vi "core_h5_write_array_3d.vi"(4 "dim3 (index)":string="index", 6 "dim2 (index)":string="index", 7 "dataset name":string, 8 "error in (no error)":errorcluster, 9 "dim1 (index)":string="index", 10 "units (au)":string="au", 11 "h5 obj ref":i32) -> (0 "error out":errorcluster, 3 "h5 obj ref":i32)   [LabVIEW 2015]
uses:
  <vilib>/addons/h5labview2/base/lib_path.vi
  <vilib>/addons/h5labview2/base/H5Equery.vi
  <vilib>/addons/h5labview2/attrib/H5Awrite.llb/H5Awrite.xnode
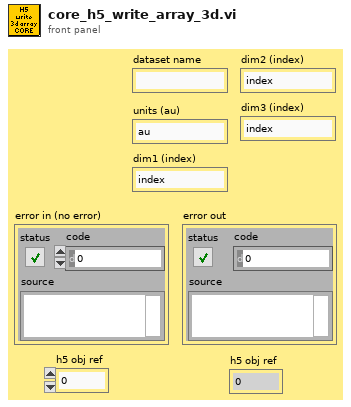
[diagram p1: front panel]
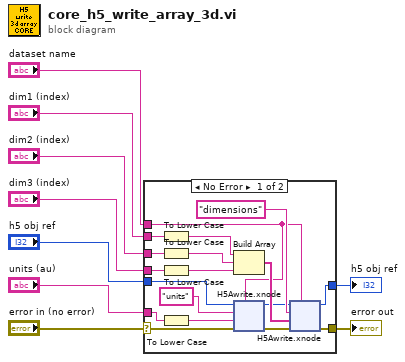
[diagram p0: block diagram]
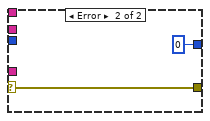
[diagram p2: hidden frame]
diagram:
  n1 = case shown="No Error" "error in (no error)" {
    selector: "error in (no error)" -> [w18 w67]
    tunnel: "h5 obj ref" -> [w19 _]
    tunnel: "dataset name" -> [w22 _]
    tunnel: [w21 w67] -> w8
    tunnel: [w20 0] -> w7
    tunnel: "dim1 (index)" -> [w17 _]
    tunnel: "dim2 (index)" -> [w15 _]
    tunnel: "units (au)" -> [w13 _]
    tunnel: "dim3 (index)" -> [w11 _]
    frame No Error {
      n2 = To Lower Case(string=w17) -> (all lower case string=w16:string)
      n3 = To Lower Case(string=w15) -> (all lower case string=w14:string)
      n4 = To Lower Case(string=w11) -> (all lower case string=w10:string)
      n5 = To Lower Case(string=w13) -> (all lower case string=w12:string)
      n6 = Build Array(w16, w14, w10) -> (w25:string[])
      n7 = xnode "H5Awrite.xnode"("object name"=w22, "error in (no error)"=w18, "data"=w12, "attrib name"="units", "ref in"=w19) -> ("error out"=w24:errorcluster, "ref out"=w23:i32)  [unwired: 2 in, 1 out]
      n8 = xnode "H5Awrite.xnode"("object name"=w22, "error in (no error)"=w24, "data"=w25, "attrib name"="dimensions", "ref in"=w23) -> ("error out"=w21:errorcluster, "ref out"=w20:i32)  [unwired: 2 in, 1 out]
    }
    frame Error {
    }
  }
  "error out" <- w8
  "h5 obj ref" <- w7
